vi "Balance_Sweep_Sever.vi"(6 "Mode":bool, 7 "Filename":string, 8 "error in":errorcluster, 9 "Sample Freq (Hz)":dbl=20000.0, 10 "Stop Angle (deg)":dbl=-2.0, 11 "Measurement Time (ms)":u32) -> (0 "error out":errorcluster)   [LabVIEW 2022 SP3]
uses:
  Gen Trav/Trav_mode.ctl
  Globals/Trav_pos_global.vi
  Globals/Meas_global.vi
  Controls/Post_Process.ctl
  <userlib>/LV-Link3/PolySubVIs/DtCreateAinChan.vi
  <userlib>/LV-Link3/PolySubVIs/DtOLReadMultiple2D.vi
  <userlib>/LV-Link3/PolySubVIs/DtOLTimingSetInput.vi
  Controls/Live Balance Data.ctl
panel:
  out "status":bool=TRUE
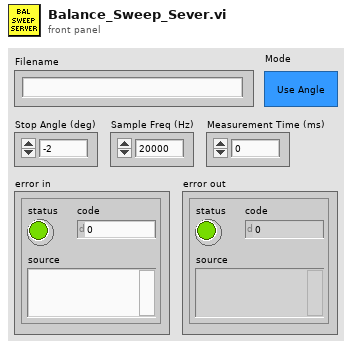
[diagram p1: front panel]
types:
  T1 = typedef "Post_Process.ctl" = enum16{"Take New Data", "Post Process Raw Data File"}
  T2 = typedef "Trav_mode.ctl" = enum16{"Move traverse", "Read traverse position", "Teach Position"}
  T3 = typedef "Live Balance Data.ctl" = cluster{"AS Freq (Hz)":dbl, "Time (s)":dbl[], "Pressure 2 (V)":dbl[], "Pressure 3 (V)":dbl[], "Wind Speed (m/s)":dbl[], "Balance AS Freq (Hz)":dbl[], "Live Angle (deg)":dbl[], "Live Angle An(deg)":dbl[], "Balance Loads":cluster{"Lift (%)":dbl[], "Lift (N)":dbl[], "Pitch (%)":dbl[], "Pitch (Nm)":dbl[], "Drag (%)":dbl[], "Drag (N)":dbl[], "Side (%)":dbl[], "Side (N)":dbl[], "Yaw (%)":dbl[], "Yaw (Nm)":dbl[], "Roll (%)":dbl[], "Roll (Nm)":dbl[]}, "Pressure 1 (V)":dbl[], "Pressure SJ (V)":dbl[]}
  T4 = enum16{"big-endian, network order", "native, host order", "little-endian"}
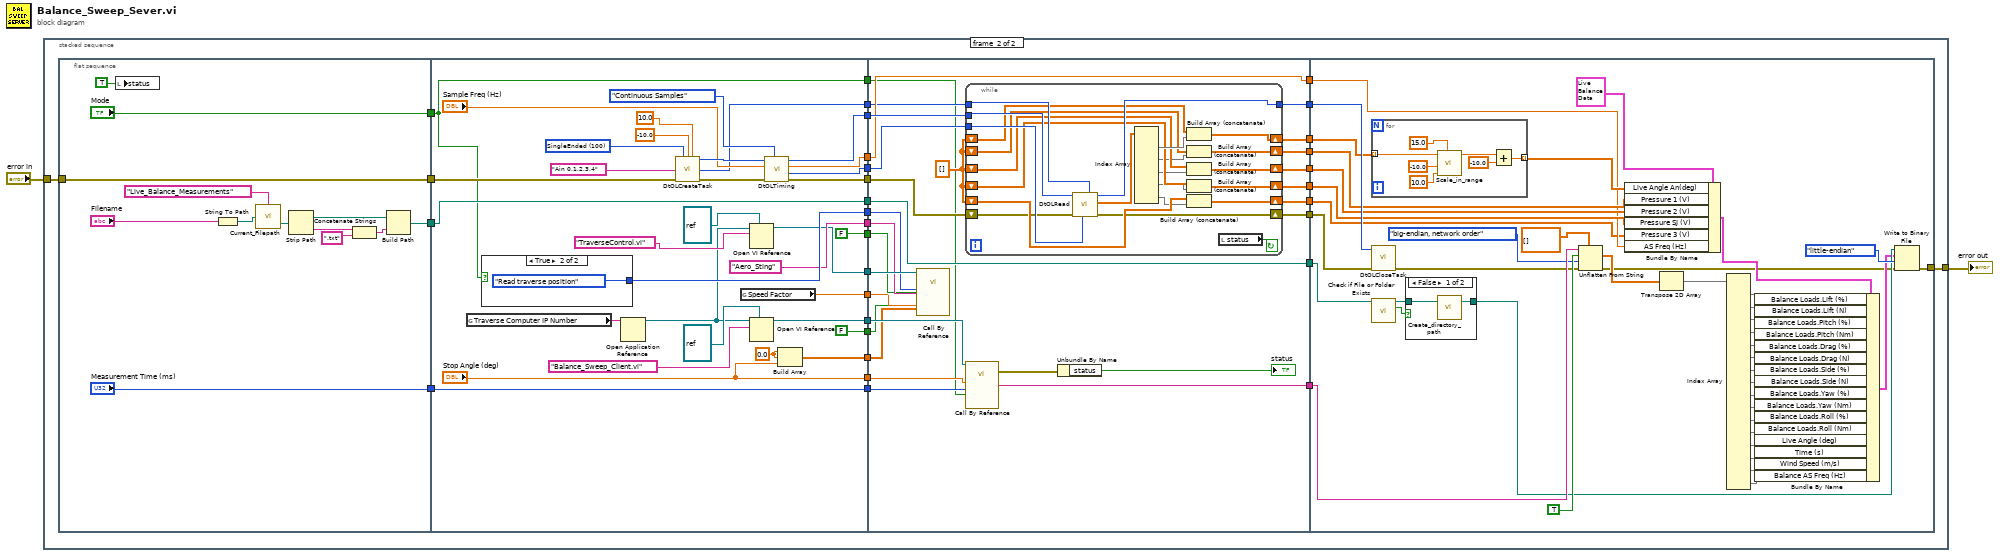
[diagram p0: block diagram]
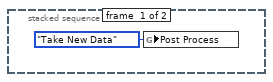
[diagram p2: hidden frame]
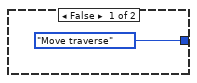
[diagram p3: hidden frame]
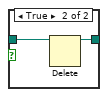
[diagram p4: hidden frame]
diagram:
  n1 = stacked-sequence {
    tunnel: [_ w12] -> w2
    tunnel: "error in" -> [_ w8]
    frame #0 {
      n2 = global write "Meas_global.vi" "Post Process"(Post_Process."Take New Data" ("Post Process")) -> ()
    }
    frame #1 {
      n3 = flat-sequence {
        tunnel: [w45] -> w36
        tunnel: [w39] -> w11
        tunnel: w8 -> [w39]
        tunnel: ["Measurement Time (ms)"] -> w7
        tunnel: ["Mode"] -> w4
        tunnel: [FALSE ("Route Checking?")] -> w35
        tunnel: [w80] -> w34
        tunnel: ["Aero_Sting" ("Traverse name")] -> w33
        tunnel: [w78] -> w32
        tunnel: [w76] -> w31
        tunnel: ["Stop Angle (deg)"] -> w30
        tunnel: [w73] -> w29
        tunnel: [w68] -> w28
        tunnel: w36 -> [w73]
        tunnel: [w67] -> w25
        tunnel: [FALSE ("Backlash Compensation?")] -> w24
        tunnel: [w58] -> w23
        tunnel: [w57] -> w22
        tunnel: [w56] -> w20
        tunnel: [w55] -> w19
        tunnel: w11 -> [w54]
        tunnel: [w52] -> w10
        tunnel: w7 -> [w51]
        tunnel: [w51] -> w6
        tunnel: [w50] -> w5
        tunnel: w4 -> [w50]
        tunnel: w35 -> [w104]
        tunnel: w34 -> [w105]
        tunnel: w33 -> [w107]
        tunnel: w32 -> [w106]
        tunnel: w31 -> [w112]
        tunnel: [w111] -> w27
        tunnel: w30 -> [w110]
        tunnel: [w109] -> w26
        tunnel: w29 -> [w109]
        tunnel: w28 -> [w108]
        tunnel: w25 -> [w103]
        tunnel: w24 -> [w102]
        tunnel: w23 -> [w101]
        tunnel: w22 -> [w100]
        tunnel: [w99] -> w21
        tunnel: w20 -> [w99]
        tunnel: w19 -> [w98]
        tunnel: [w97] -> w18
        tunnel: [w95] -> w17
        tunnel: [w94] -> w16
        tunnel: [w93] -> w15
        tunnel: [w92] -> w14
        tunnel: [w90] -> w13
        tunnel: w10 -> [w88]
        tunnel: [w87] -> w9
        tunnel: w6 -> [w86]
        tunnel: w5 -> [w85]
        tunnel: w27 -> [w172]
        tunnel: w26 -> [w177]
        tunnel: w21 -> [w141]
        tunnel: w18 -> [w168]
        tunnel: w17 -> [w143]
        tunnel: w16 -> [w146]
        tunnel: w15 -> [w145]
        tunnel: w14 -> [w144]
        tunnel: w13 -> [w140]
        tunnel: [w139] -> w12
        tunnel: w9 -> [w138]
        frame #0 {
          n4 = local write "status"(TRUE ("status")) -> ()
          n5 = String To Path(string="Filename") -> (path=w47:path)
          n6 = call "Current_Filepath.vi"("Filename in"=w47, "Data Type"="Live_Balance_Measurements") -> ("Filename Out"=w48:path)  [unwired: 1 out]
          n7 = Strip Path(path=w48) -> (stripped path=w41:path, name=w44:string)
          n8 = Concatenate Strings(w44, ".txt" ("string")) -> (w42:string)
          n9 = Build Path(base path=w41, name or relative path=w42) -> (appended path=w45:path)
        }
        frame #1 {
          w62 = 100 items=["SingleEnded"=100, "Differential"=101] ("Channel Type")
          w82 = 0.0
          n10 = global read "Trav_pos_global.vi" "Traverse Computer IP Number"() -> (w72:string)
          n11 = case shown="True" w50 {
            tunnel: [Trav_mode."Move traverse" ("Mode") Trav_mode."Read traverse position" ("Mode")] -> w80
            frame False {
            }
            frame True {
            }
          }
          n12 = Open Application Reference(11:w72) -> (3:w69:refnum<vi>)  [unwired: 3 in, 1 out]
          n13 = call-poly <userlib>:"DtOLCreateTask.vi"("Channel Type"=w62, "Range Min"=-10.0, "Range Max"=10.0, "Channel"="Ain 0,1,2,3,4", "error in (no error)"=w54) -> ("Task out"=w61:i32, "Actual Number of Channels"=w55:u32, "error out"=w53:errorcluster)  [unwired: 8 in]
          n14 = global read "Trav_pos_global.vi" "Speed Factor"() -> (w67:sgl)
          n15 = Open VI Reference(type specifier VI Refnum (for type only)=refnum<vi> refnum, application reference (local)=w69, vi path="TraverseControl.vi" ("Traverse name")) -> (vi reference=w68:refnum<vi>)  [unwired: 3 in, 1 out]
          n16 = Open VI Reference(type specifier VI Refnum (for type only)=refnum<vi> refnum, application reference (local)=w69, vi path="Balance_Sweep_Client.vi" ("Traverse name")) -> (vi reference=w76:refnum<vi>)  [unwired: 3 in, 1 out]
          n17 = call-poly <userlib>:"DtOLTiming.vi"("Sample Mode"=enum16{"Finite Samples", "Continuous Samples"}."Continuous Samples", "error in (no error)"=w53, "Sample Freq (Hz)"="Sample Freq (Hz)", "Task in"=w61) -> ("error out"=w52:errorcluster, "Buffer Size"=w58:u32, "Actual Sample Freq"=w56:dbl, "Task out"=w57:i32)  [unwired: 4 in]
          n18 = Build Array(w82, w82, "Stop Angle (deg)") -> (w78:dbl[])
        }
        frame #2 {
          w91 = dbl[] []
          n19 = call-by-ref "?"(reference=w108, "Mode"=w105, "Route Checking?"=w104, "Traverse Name"=w107, "Position input XYZ"=w106, "Speed Factor"=w103, "Backlash Compensation?"=w102) -> ()  [unwired: 9 in, 4 out]
          n20 = while {
            tunnel: w101 -> [w135]
            tunnel: w100 -> [w134]
            tunnel: w98 -> [w133]
            tunnel: [w132] -> w97
            shift-right: [w127] -> w95
            shift-left: w91 -> [w128]
            shift-right: [w126] -> w94
            shift-left: w91 -> [w125]
            shift-right: [w123] -> w93
            shift-left: w91 -> [w124]
            shift-right: [w117] -> w92
            shift-left: w91 -> [w122]
            shift-right: [w115] -> w90
            shift-left: w91 -> [w118]
            shift-right: [w113] -> w87
            shift-left: w88 -> [w114]
            stop <- w131 continue-if-true
            n21 = call-poly <userlib>:"DtOLRead.vi"("Number Chan to Read"=w133, "Buffer size"=w135, "error in (no error)"=w114, "Task in"=w134) -> ("error out"=w113:errorcluster, "2D Data out"=w130:dbl[][], "Task out"=w132:i32)  [unwired: 3 in, 2 out]
            n22 = Index Array(array=w130) -> (element #1=w129:dbl[], element #2=w121:dbl[], element #3=w120:dbl[], element #4=w119:dbl[], element #5=w116:dbl[])  [unwired: 10 in]
            n23 = Build Array (concatenate)(w128, w129) -> (w127:dbl[])
            n24 = Build Array (concatenate)(w125, w121) -> (w126:dbl[])
            n25 = Build Array (concatenate)(w124, w120) -> (w123:dbl[])
            n26 = Build Array (concatenate)(w122, w119) -> (w117:dbl[])
            n27 = Build Array (concatenate)(w118, w116) -> (w115:dbl[])
            n28 = local read "status"() -> (w131:bool)
          }
          n29 = call-by-ref "?"(reference=w112, "Mode"=w85, "Measurement Time (ms)"=w86, "Stop Angle"=w110) -> (error out=w96:errorcluster, "Data Out"=w111:string)  [unwired: 3 in, 1 out]
          n30 = Unbundle By Name(w96) -> ("status"=→"status":bool)
        }
        frame #3 {
          n31 = for {
            tunnel: [w181] -> w142 mode=indexing
            tunnel: w143 -> [w178] mode=indexing
            n32 = call "Scale_in_range.vi"("Scale Factor"=15.0, "Maximum Range"=10.0, "Minimum Range"=-10.0, "x"=w178) -> ("Scaled x"=w183:dbl)  [unwired: 7 in]
            n33 = Add(x=w183, y=-10.0) -> (x+y=w181:dbl)
          }
          n34 = call <userlib>:"DtOLCloseTask.vi"("Error in"=w138, "Task in"=w168) -> ("Error Out"=w137:errorcluster)  [unwired: 9 in]
          n35 = call <vilib>:"Check if File or Folder Exists.vi"("path"=w177) -> ("file or folder exists?"=w176:bool, "dup path"=w175:path)  [unwired: 8 in, 1 out]
          n36 = case shown="False" w176 {
            tunnel: w175 -> [w186 w188]
            tunnel: [w185 w187] -> w169
            frame False {
              n37 = call "Create_directory_path.vi"("Path name"=w186) -> ("Path name Out"=w185:path)  [unwired: 1 in, 1 out]
            }
            frame True {
              n38 = Delete(path (use dialog)=w188) -> (deleted path=w187:path)  [unwired: 4 in, 2 out]
            }
          }
          n39 = Unflatten From String(type=dbl[][] [], binary string=w172, data includes array or string size? (T)=TRUE, byte order (0:big-endian, network order)=T4."big-endian, network order", error in (no error)=w137) -> (value=w166:dbl[][], error out=w136:errorcluster)  [unwired: 1 out]
          n40 = Bundle By Name(cluster=T3 {"AS Freq (Hz)"=0.0, "Time (s)"=[], "Pressure 2 (V)"=[], "Pressure 3 (V)"=[], "Wind Speed (m/s)"=[], "Balance AS Freq (Hz)"=[], "Live Angle (deg)"=[], "Live Angle An(deg)"=[], "Balance Loads"={"Lift (%)"=[], "Lift (N)"=[], "Pitch (%)"=[], "Pitch (Nm)"=[], "Drag (%)"=[], "Drag (N)"=[], "Side (%)"=[], "Side (N)"=[], "Yaw (%)"=[], "Yaw (Nm)"=[], "Roll (%)"=[], "Roll (Nm)"=[]}, "Pressure 1 (V)"=[], "Pressure SJ (V)"=[]} ("input cluster"), "Live Angle An(deg)"=w142, "Pressure 1 (V)"=w146, "Pressure 2 (V)"=w145, "Pressure SJ (V)"=w144, "Pressure 3 (V)"=w140, "AS Freq (Hz)"=w141) -> (w165:T3)
          n41 = Transpose 2D Array(2D array=w166) -> (transposed array=w164:dbl[][])
          n42 = Index Array(array=w164) -> (element #1=w162:dbl[], element #2=w161:dbl[], element #3=w160:dbl[], element #4=w159:dbl[], element #5=w158:dbl[], element #6=w157:dbl[], element #7=w156:dbl[], element #8=w155:dbl[], element #9=w154:dbl[], element #10=w153:dbl[], element #11=w152:dbl[], element #12=w151:dbl[], element #13=w150:dbl[], element #14=w149:dbl[], element #15=w148:dbl[], element #16=w147:dbl[])  [unwired: 32 in]
          n43 = Bundle By Name(cluster=w165, "Balance Loads.Lift (%)"=w162, "Balance Loads.Lift (N)"=w161, "Balance Loads.Pitch (%)"=w160, "Balance Loads.Pitch (Nm)"=w159, "Balance Loads.Drag (%)"=w158, "Balance Loads.Drag (N)"=w157, "Balance Loads.Side (%)"=w156, "Balance Loads.Side (N)"=w155, "Balance Loads.Yaw (%)"=w154, "Balance Loads.Yaw (Nm)"=w153, "Balance Loads.Roll (%)"=w152, "Balance Loads.Roll (Nm)"=w151, "Live Angle (deg)"=w150, "Time (s)"=w149, "Wind Speed (m/s)"=w148, "Balance AS Freq (Hz)"=w147) -> (w163:T3)
          n44 = Write to Binary File(file (use dialog)=w169, data=w163, error in=w136, 9:T4."little-endian" ("byte order (0:big-endian, network order)")) -> (error out=w139:errorcluster)  [unwired: 2 in, 2 out]
        }
      }
    }
  }
  "error out" <- w2
